vi "CLAD Exercise 3-6.vi"() -> ()   [LabVIEW 2014]
panel:
  out "Result":dbl
  out "Result":dbl
  in  "Fahrenheit":bool
  in  "Celsius":bool
  in  "Temperature (C)":dbl
  in  "Temperature (F)":dbl
  # "Kelvin"
  # "Kelvin"
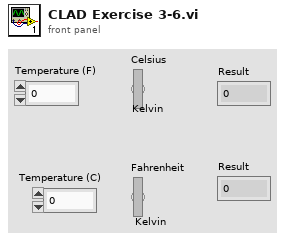
[diagram p1: front panel]
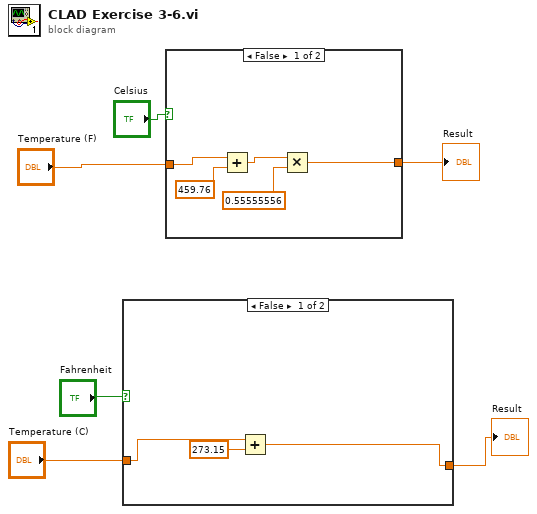
[diagram p0: block diagram]
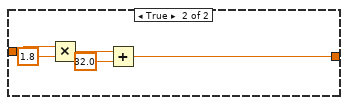
[diagram p2: hidden frame]
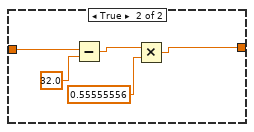
[diagram p3: hidden frame]
diagram:
  n1 = case shown="False" "Fahrenheit" {
    tunnel: "Temperature (C)" -> [w9 w14]
    tunnel: [w7 w10] -> w1
    frame False {
      n2 = Add(x=w9, y=273.15) -> (x+y=w7:dbl)
    }
    frame True {
      n3 = Multiply(x=w14, y=1.8) -> (x*y=w12:dbl)
      n4 = Add(x=w12, y=32.0) -> (x+y=w10:dbl)
    }
  }
  "Result" <- w1
  n5 = case shown="False" "Celsius" {
    tunnel: "Temperature (F)" -> [w19 w24]
    tunnel: [w15 w20] -> w4
    frame False {
      n6 = Add(x=w19, y=459.76) -> (x+y=w17:dbl)
      n7 = Multiply(x=w17, y=0.55555556) -> (x*y=w15:dbl)
    }
    frame True {
      n8 = Subtract(x=w24, y=32.0) -> (x-y=w22:dbl)
      n9 = Multiply(x=w22, y=0.55555556) -> (x*y=w20:dbl)
    }
  }
  "Result" <- w4
